vi "Boiler.vi"() -> ()   [LabVIEW 2020]
doc: "The VI \"Boiler\" is designed to simulate the operation of a boiler startup controller. This VI uses a state machine to control the states of its execution sequentially. Outside of the state machine are input variables that determine the maximum and minimum values required for events to take place as well the ability to name the event log file. Each state is indicated by the Boiler Status Indicators on the Front Panel and data collected from each state is written to the event log file. The states (with a short description of how to get to each state when applicable) are as follows and will repeat until the user presses STOP:\n\n1) Reset Controls and Indicators\n If state 10 has been executed: Wait 10s (or inputted value) for Shutdown and Purge to complete\n2) Start (Application Run)\n3) Reset Lockout\n \"Run Interlock\" ON and\n \"Boiler Reset\" ON\n4) Pre-Purge\n \"Start Sequence\" is ON\n5) Pre-Purge (continued)\n Wait 10 s (or inputted value) for Pre-Purge to complete\n6) Ignition (Ignite Pilot)\n \"Pilot\" is ON\n7) Prove the Pilot\n Flame Sensor Value (%) > 30 (or inputted minimum value)\n8) Start and Run\n Forced Draft Fan ON\n9) Start and run (continued)\n Fuel Valve Position > 10 (or inputted minimum value)\n10) Shutdown and Purge\n Run Interlock OFF or\n Forced Draft Fan OFF or\n Shutdown ON or\n Fuel Valve Position > 75 (or inputted maximum value) or\n Fuel Valve Position < 10 (or inputted minimum value)"
uses:
  Controls/Boiler Controls.ctl
  Controls/Boiler Simulation Controls.ctl
  Controls/Boiler Status Indicators.ctl
  Boiler States.ctl
panel:
  in  "stop":bool
  out "Boiler Status Indicators":T1 {"Time Count" format="%.2g"}
  in  "Boiler Simulation Controls":T2 {"Flame Sensor Value (%)" min=0.0 max=100.0 scale=0.0..100.0}
  in  "Boiler Controls":T3 {"Fuel Valve Position" min=0.0 max=100.0 scale=0.0..100.0 scale format="%.2f"}
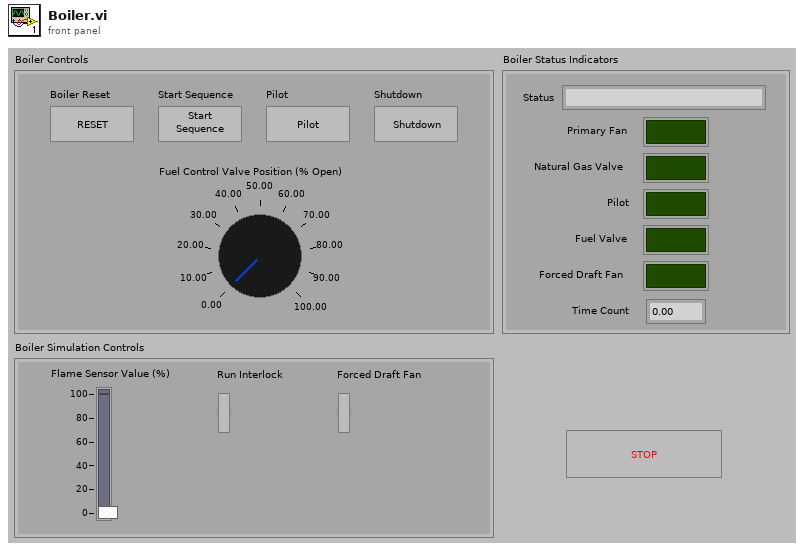
[diagram p1: front panel]
types:
  T1 = typedef "Boiler Status Indicators.ctl" = cluster{"Status":string, "Primary Fan":bool, "Natural Gas Valve":bool, "Pilot":bool, "Fuel Valve":bool, "Forced Draft Fan":bool, "Time Count":dbl}
  T2 = typedef "Boiler Simulation Controls.ctl" = cluster{"Flame Sensor Value (%)":dbl, "Run Interlock":bool, "Forced Draft Fan":bool}
  T3 = typedef "Boiler Controls.ctl" = cluster{"Boiler Reset":bool, "Start Sequence":bool, "Pilot":bool, "Shutdown":bool, "Fuel Valve Position":dbl}
  T4 = typedef "Boiler States.ctl" = enum16{"Reset Controls and Indicators", "Start (Application Run)", "Reset Lockout", "Pre-Purge", "Pre-Purge (continued)", "Ignition (Ignite Pilot)", "Prove the Pilot", "Start and Run", "Start and Run (continued)", "Shutdown and Purge"}
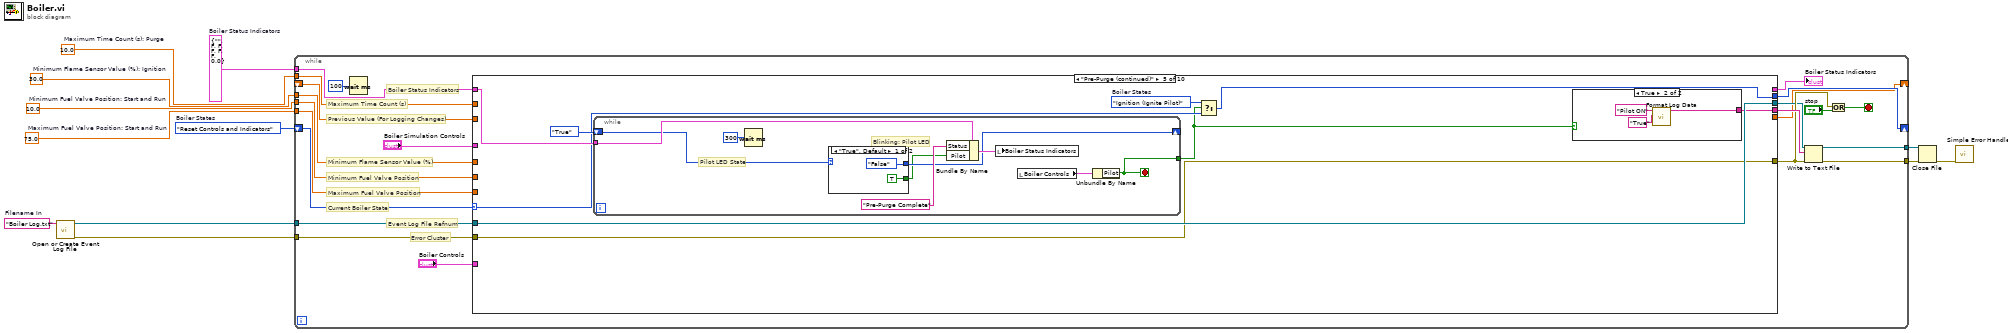
[diagram p0: block diagram]
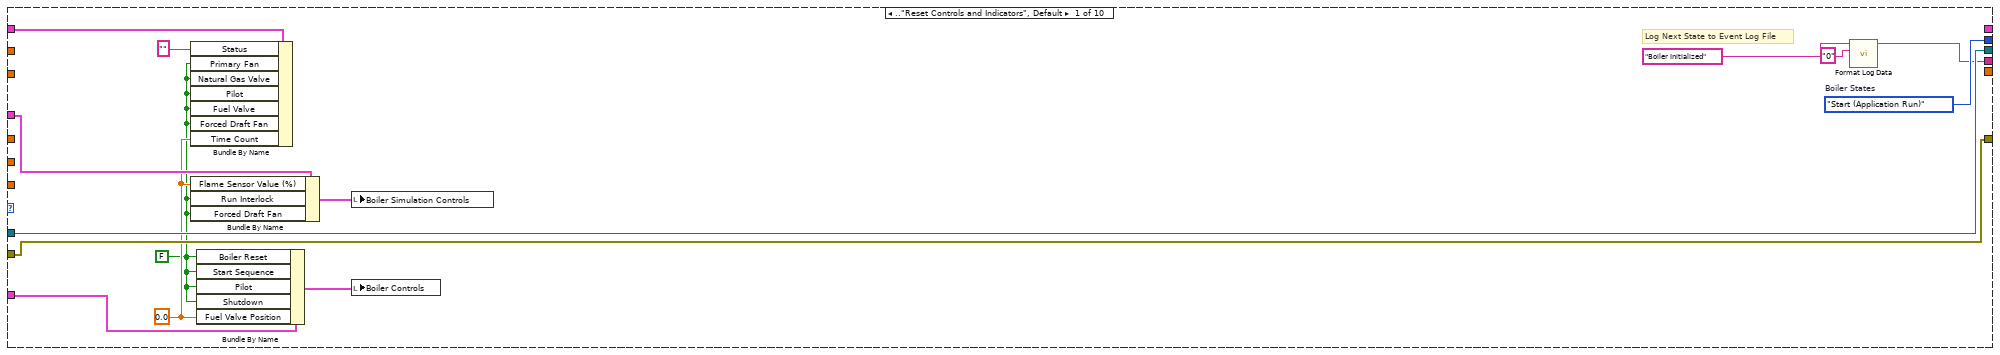
[diagram p2: hidden frame]
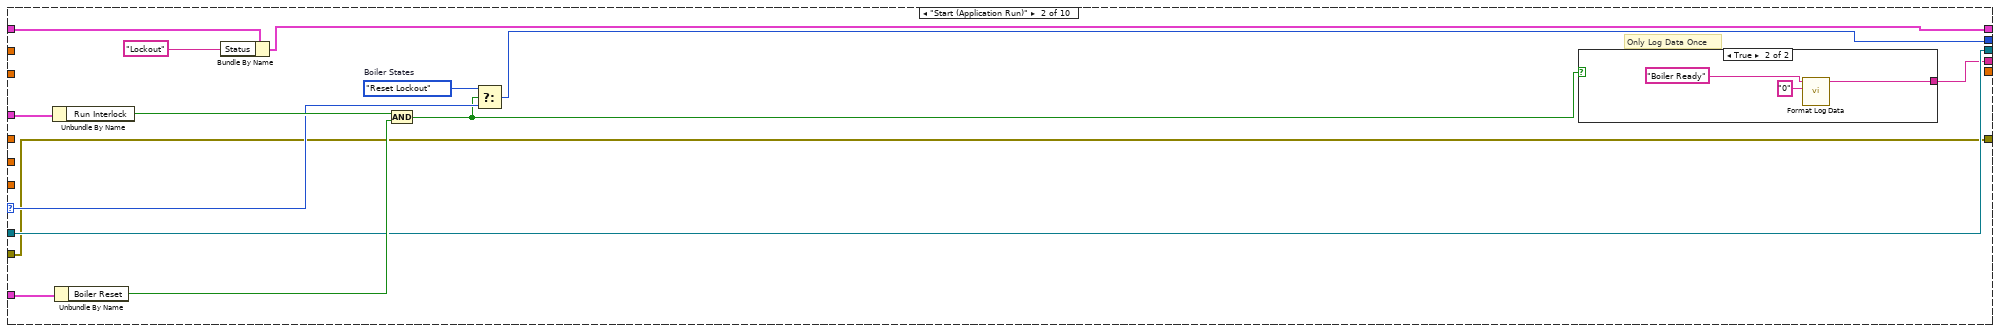
[diagram p3: hidden frame]
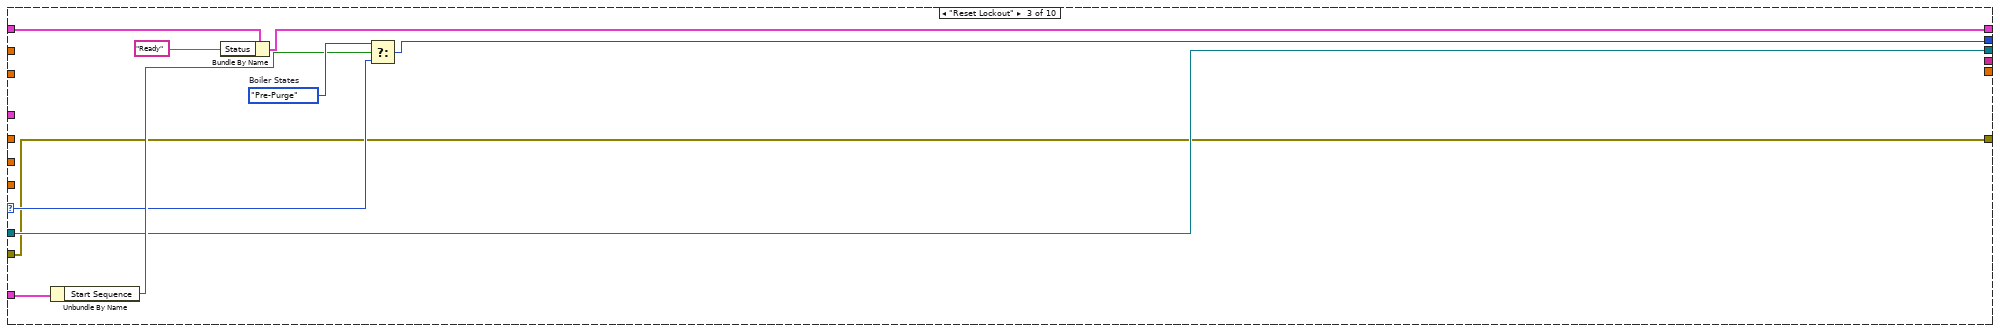
[diagram p5: hidden frame]
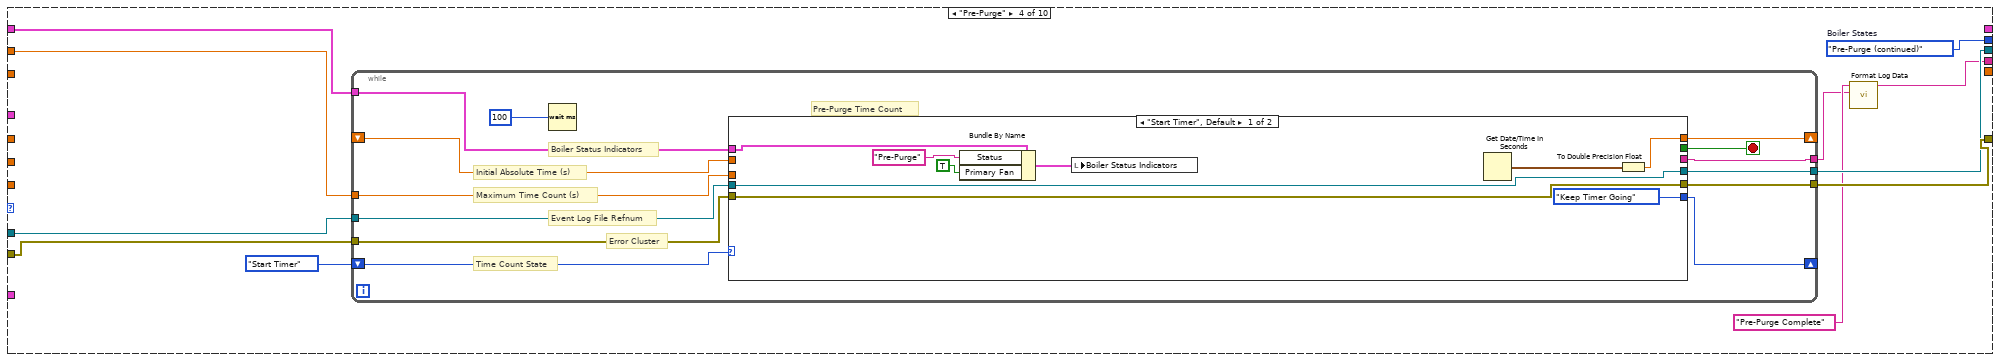
[diagram p6: hidden frame]
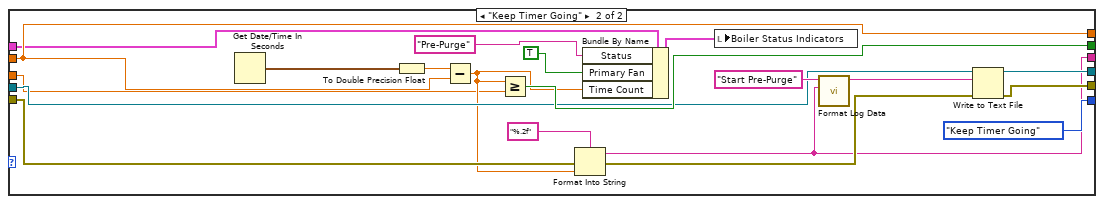
[diagram p7: hidden frame]
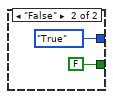
[diagram p9: hidden frame]
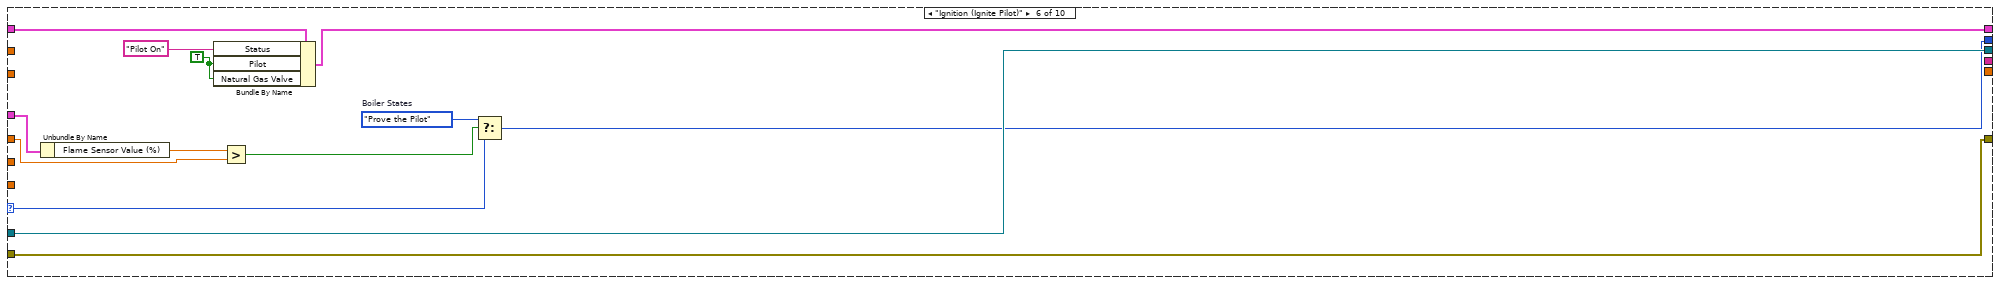
[diagram p10: hidden frame]
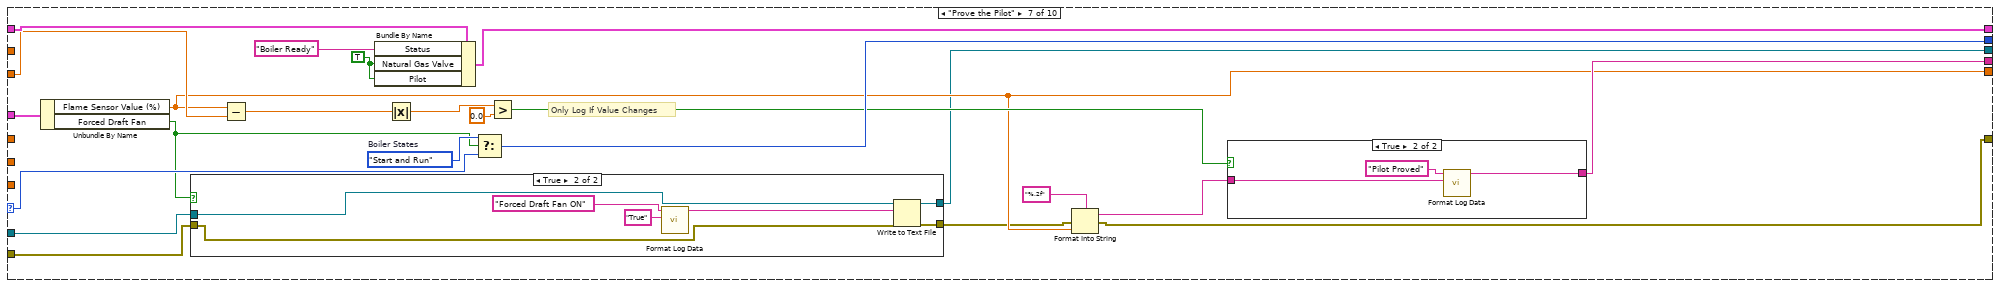
[diagram p11: hidden frame]
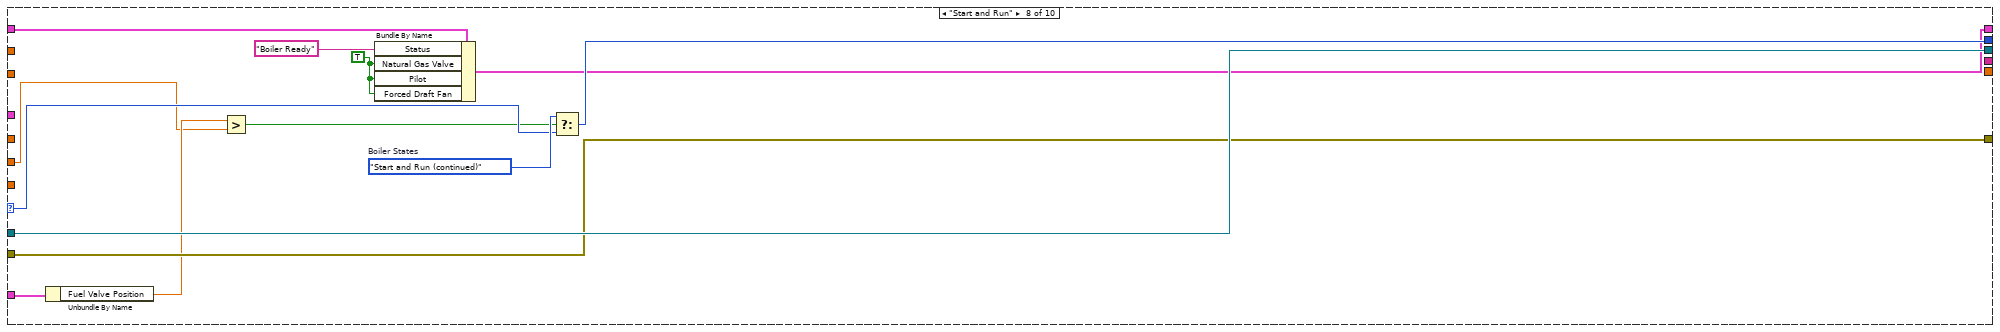
[diagram p14: hidden frame]
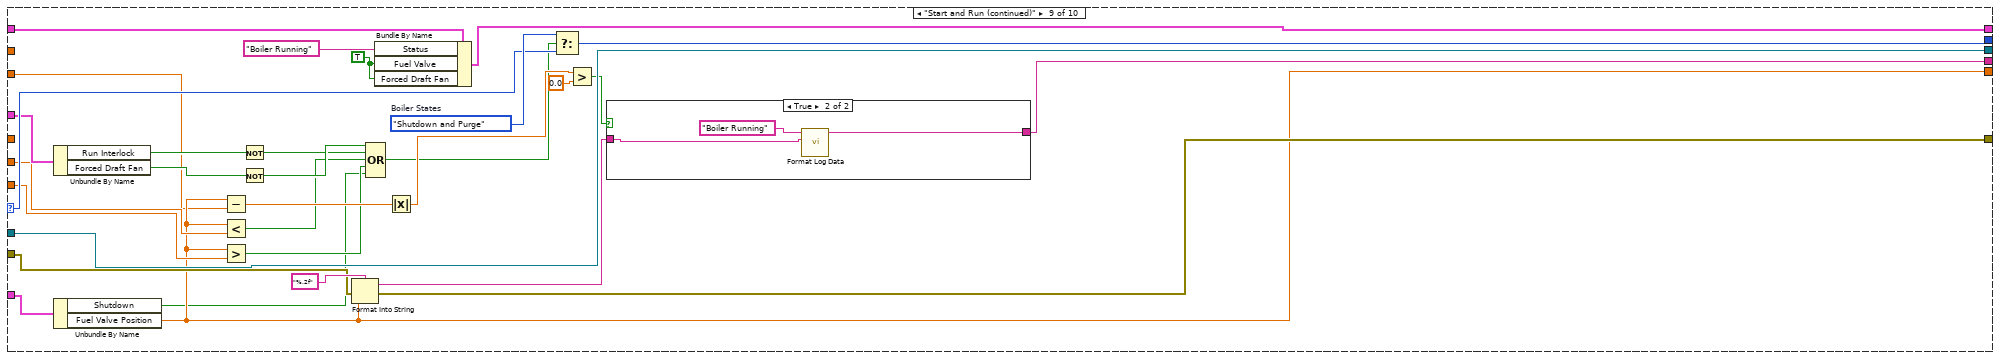
[diagram p15: hidden frame]
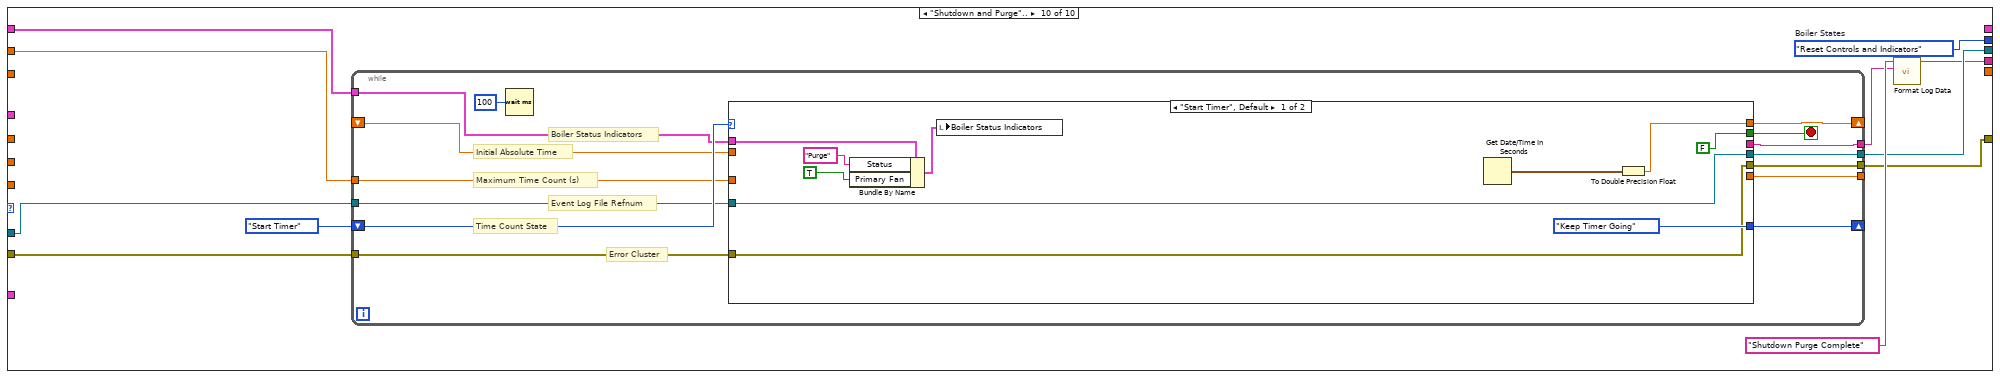
[diagram p17: hidden frame]
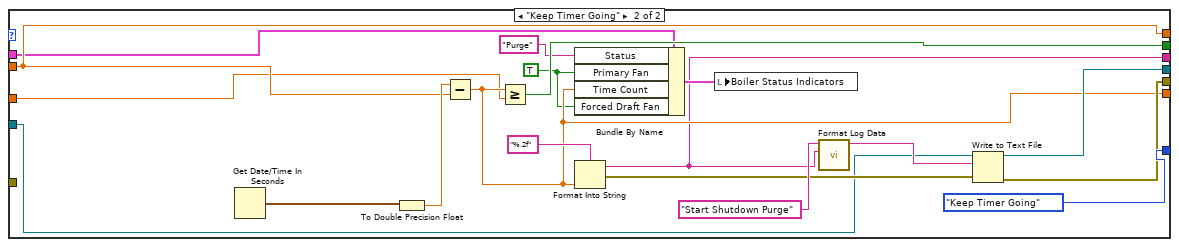
[diagram p18: hidden frame]
diagram:
  w1 = 75.0  # Maximum Fuel Valve Position: Start and Run
  w2 = 10.0  # Minimum Fuel Valve Position: Start and Run
  w3 = 30.0  # Minimum Flame Sensor Value (%): Ignition
  w4 = 10.0  # Maximum Time Count (s): Purge
  w5 = "Boiler Log.txt"  # Filename In
  w12 = T1 {"Status"="", "Primary Fan"=FALSE, "Natural Gas Valve"=FALSE, "Pilot"=FALSE, "Fuel Valve"=FALSE, "Forced Draft Fan"=FALSE, "Time Count"=0.0}  # Boiler Status Indicators
  w6 = Boiler_States."Reset Controls and Indicators"  # Boiler States
  n1 = call "Open or Create Event Log File.vi"("Filename In"=w5) -> ("error out"=w7:errorcluster, "refnum out"=w8:refnum<file>)  [unwired: 9 in]
  n2 = while {
    tunnel: w12 -> [w19]
    tunnel: [w29] -> w11
    tunnel: [w28] -> w10
    shift-right: [w27] -> _
    shift-left: w6 -> [w33]
    tunnel: w8 -> [w21]
    tunnel: w7 -> [w22]
    tunnel: w4 -> [w18]
    tunnel: w3 -> [w17]
    tunnel: w2 -> [w16]
    tunnel: w1 -> [w15]
    shift-right: [w14] -> _
    shift-left: _ -> [w13]
    stop <- w25 stop-if-true
    # "Previous Value (For Logging Changes)"
    # "Maximum Fuel Valve Position"
    # "Minimum Fuel Valve Position"
    # "Minimum Flame Sensor Value (%)"
    # "Maximum Time Count (s)"
    # "Boiler Status Indicators"
    # "Error Cluster"
    # "Event Log File Refnum"
    # "Current Boiler State"
    n3 = Wait (ms)(milliseconds to wait=u32 100) -> ()  [unwired: 1 out]
    n4 = case shown="\"Pre-Purge (continued)\"" w33 {
      selector: w33 -> [_ w53 w68 _ w135 w159 w180 w212 w234 _]
      tunnel: "Boiler Simulation Controls" -> [w45 w58 _ _ _ w157 w185 _ w233 _]
      tunnel: "Boiler Controls" -> [w43 w56 w70 _ _ _ _ w208 w232 _]
      tunnel: [_ w61 w74 _ _ w165 w189 w202 w244 _] -> w30
      tunnel: w19 -> [w41 w62 w75 w81 w137 w166 w188 w214 w245 w258]
      tunnel: [w48 w54 w71 w80 w133 w158 w179 w211 w235 w257] -> w27
      tunnel: [w35 w49 _ w77 w129 _ w186 _ w242 w251] -> w24
      tunnel: [w46 w51 w66 w85 w131 w162 w183 w209 w238 w253] -> w23
      tunnel: w22 -> [w46 w51 w66 w84 w131 w162 w170 w209 w239 w254]
      tunnel: w21 -> [w47 w52 w67 w83 w132 w161 w169 w210 w241 w255]
      tunnel: [w47 w52 w67 w82 w132 w161 w168 w210 w241 w252] -> w20
      tunnel: w18 -> [_ _ _ w76 _ _ _ _ _ w249]
      tunnel: w17 -> [_ _ _ _ _ w154 _ _ _ _]
      tunnel: w16 -> [_ _ _ _ _ _ _ w203 w228 _]
      tunnel: w15 -> [_ _ _ _ _ _ _ _ w227 _]
      tunnel: [_ _ _ _ _ _ w172 _ w226 _] -> w14
      tunnel: w13 -> [_ _ _ _ _ _ w173 _ w225 _]
      frame .."Reset Controls and Indicators", Default {
        w38 = FALSE ("Run Interlock")
        w39 = 0.0 ("Flame Sensor Value (%)")
        w48 = Boiler_States."Start (Application Run)"  # Boiler States
        # "Log Next State to Event Log File"
        n5 = Bundle By Name(cluster=w41, "Status"="", "Primary Fan"=w38, "Natural Gas Valve"=w38, "Pilot"=w38, "Fuel Valve"=w38, "Forced Draft Fan"=w38, "Time Count"=w39) -> ()  [unwired: 1 out]
        n6 = Bundle By Name(cluster=w45, "Flame Sensor Value (%)"=w39, "Run Interlock"=w38, "Forced Draft Fan"=w38) -> (w44:T2)
        n7 = Bundle By Name(cluster=w43, "Boiler Reset"=w38, "Start Sequence"=w38, "Pilot"=w38, "Shutdown"=w38, "Fuel Valve Position"=w39) -> (w42:T3)
        n8 = local write "Boiler Simulation Controls"(w44) -> ()
        n9 = local write "Boiler Controls"(w42) -> ()
        n10 = call "Format Log Data.vi"("Event Data String:"="0", "Event String:"="Boiler Initialized") -> ("Formatted Log Data"=w35:string)  [unwired: 9 in]
      }
      frame "Start (Application Run)" {
        w59 = Boiler_States."Reset Lockout"  # Boiler States
        # "Only Log Data Once"
        n11 = Unbundle By Name(w58) -> ("Run Interlock"=w57:bool)
        n12 = Unbundle By Name(w56) -> ("Boiler Reset"=w55:bool)
        n13 = Bundle By Name(cluster=w62, "Status"="Lockout") -> (w61:T1)
        n14 = And(x=w57, y=w55) -> (x .and. y?=w50:bool)
        n15 = Select(t=w59, s=w50, f=w53) -> (s? t:f=w54:T4)
        n16 = case shown="True" w50 {
          tunnel: [_ w63] -> w49
          frame False {
          }
          frame True {
            n17 = call "Format Log Data.vi"("Event Data String:"="0", "Event String:"="Boiler Ready") -> ("Formatted Log Data"=w63:string)  [unwired: 9 in]
          }
        }
      }
      frame "Reset Lockout" {
        w72 = Boiler_States."Pre-Purge"  # Boiler States
        n18 = Unbundle By Name(w70) -> ("Start Sequence"=w69:bool)
        n19 = Bundle By Name(cluster=w75, "Status"="Ready") -> (w74:T1)
        n20 = Select(t=w72, s=w69, f=w68) -> (s? t:f=w71:T4)
      }
      frame "Pre-Purge" {
        w80 = Boiler_States."Pre-Purge (continued)"  # Boiler States
        n21 = while {
          tunnel: w81 -> [w99]
          shift-right: [w96] -> _
          shift-left: enum16{"Start Timer", "Keep Timer Going"}."Start Timer" -> [w97]
          shift-right: [w95] -> _
          shift-left: _ -> [w94]
          tunnel: [w92] -> w85
          tunnel: w84 -> [w91]
          tunnel: w83 -> [w90]
          tunnel: [w89] -> w82
          tunnel: [w88] -> w78
          tunnel: w76 -> [w87]
          stop <- w93 stop-if-true
          # "Pre-Purge Time Count"
          # "Maximum Time Count (s)"
          # "Boiler Status Indicators"
          # "Initial Absolute Time (s)"
          # "Error Cluster"
          # "Time Count State"
          # "Event Log File Refnum"
          n22 = Wait (ms)(milliseconds to wait=u32 100) -> ()  [unwired: 1 out]
          n23 = case shown="\"Start Timer\", Default" w97 {
            tunnel: w99 -> [w101 w114]
            tunnel: [enum16{"Start Timer", "Keep Timer Going"}."Keep Timer Going" enum16{"Start Timer", "Keep Timer Going"}."Keep Timer Going"] -> w96
            tunnel: [w106 w124] -> w95
            tunnel: w94 -> [_ w124]
            tunnel: [_ w125] -> w93
            tunnel: [w104 w120] -> w92
            tunnel: w91 -> [w104 w117]
            tunnel: w90 -> [w105 w119]
            tunnel: [w105 w118] -> w89
            tunnel: [_ w110] -> w88
            tunnel: w87 -> [_ w109]
            frame "Start Timer", Default {
              n24 = Bundle By Name(cluster=w101, "Status"="Pre-Purge", "Primary Fan"=TRUE) -> (w100:T1)
              n25 = local write "Boiler Status Indicators"(w100) -> ()
              n26 = Get Date/Time In Seconds() -> (seconds since 1Jan1904=w107:timestamp)
              n27 = To Double Precision Float(number=w107) -> (double precision float=w106:dbl)
            }
            frame "Keep Timer Going" {
              n28 = Get Date/Time In Seconds() -> (seconds since 1Jan1904=w127:timestamp)
              n29 = To Double Precision Float(number=w127) -> (double precision float=w126:dbl)
              n30 = Subtract(x=w126, y=w124) -> (x-y=w111:dbl)
              n31 = Greater Or Equal?(x=w111, y=w109) -> (x >= y?=w125:bool)
              n32 = Format Into String "Format Into String"(format string="%.2f", error in=w117, w111) -> (resulting string=w110:string, error out=w116:errorcluster)  [unwired: 1 in]
              n33 = Bundle By Name(cluster=w114, "Status"="Pre-Purge", "Primary Fan"=TRUE, "Time Count"=w111) -> (w128:T1)
              n34 = local write "Boiler Status Indicators"(w128) -> ()
              n35 = call "Format Log Data.vi"("Event Data String:"=w110, "Event String:"="Start Pre-Purge") -> ("Formatted Log Data"=w121:string)  [unwired: 9 in]
              n36 = Write to Text File(file (use dialog)=w119, text=w121, error in=w116) -> (refnum out=w118:refnum<file>, error out=w120:errorcluster)  [unwired: 1 in, 1 out]
            }
          }
        }
        n37 = call "Format Log Data.vi"("Event Data String:"=w78, "Event String:"="Pre-Purge Complete") -> ("Formatted Log Data"=w77:string)  [unwired: 9 in]
      }
      frame "Pre-Purge (continued)" {
        w134 = Boiler_States."Ignition (Ignite Pilot)"  # Boiler States
        n38 = while {
          tunnel: w137 -> [w148]
          shift-right: [w144] -> _
          shift-left: enum16{"False", "True"}."True" -> [w145]
          tunnel: [w141] -> w130
          stop <- w141 stop-if-true
          # "Pilot LED State"
          # "Blinking: Pilot LED"
          n39 = Wait (ms)(milliseconds to wait=u32 300) -> ()  [unwired: 1 out]
          n40 = case shown="\"True\", Default" w145 {
            tunnel: [enum16{"False", "True"}."False" enum16{"False", "True"}."True"] -> w144
            tunnel: [TRUE FALSE] -> w143
            frame "True", Default {
            }
            frame "False" {
            }
          }
          n41 = Bundle By Name(cluster=w148, "Status"="Pre-Purge Complete", "Pilot"=w143) -> (w147:T1)
          n42 = local write "Boiler Status Indicators"(w147) -> ()
          n43 = local read "Boiler Controls"() -> (w142:T3)
          n44 = Unbundle By Name(w142) -> ("Pilot"=w141:bool)
        }
        n45 = Select(t=w134, s=w130, f=w135) -> (s? t:f=w133:T4)
        n46 = case shown="True" w130 {
          tunnel: [_ w138] -> w129
          frame False {
          }
          frame True {
            n47 = call "Format Log Data.vi"("Event Data String:"="True", "Event String:"="Pilot ON") -> ("Formatted Log Data"=w138:string)  [unwired: 9 in]
          }
        }
      }
      frame "Ignition (Ignite Pilot)" {
        w160 = Boiler_States."Prove the Pilot"  # Boiler States
        w163 = TRUE ("Natural Gas Valve")
        n48 = Unbundle By Name(w157) -> ("Flame Sensor Value (%)"=w156:dbl)
        n49 = Bundle By Name(cluster=w166, "Status"="Pilot On", "Pilot"=w163, "Natural Gas Valve"=w163) -> (w165:T1)
        n50 = Greater?(x=w156, y=w154) -> (0:w155:bool)
        n51 = Select(t=w160, s=w155, f=w159) -> (s? t:f=w158:T4)
      }
      frame "Prove the Pilot" {
        w178 = TRUE ("Natural Gas Valve")
        w181 = Boiler_States."Start and Run"  # Boiler States
        # "Only Log If Value Changes"
        n52 = Unbundle By Name(w185) -> ("Flame Sensor Value (%)"=w172:dbl, "Forced Draft Fan"=w171:bool)
        n53 = case shown="True" w171 {
          tunnel: w170 -> [w191 w196]
          tunnel: w169 -> [w190 w194]
          tunnel: [w190 w193] -> w168
          tunnel: [w191 w192] -> w167
          frame False {
          }
          frame True {
            n54 = call "Format Log Data.vi"("Event Data String:"="True", "Event String:"="Forced Draft Fan ON") -> ("Formatted Log Data"=w195:string)  [unwired: 9 in]
            n55 = Write to Text File(file (use dialog)=w194, text=w195, error in=w196) -> (refnum out=w193:refnum<file>, error out=w192:errorcluster)  [unwired: 1 in, 1 out]
          }
        }
        n56 = Subtract(x=w172, y=w173) -> (x-y=w177:dbl)
        n57 = Bundle By Name(cluster=w188, "Status"="Boiler Ready", "Natural Gas Valve"=w178, "Pilot"=w178) -> (w189:T1)
        n58 = Absolute Value(x=w177) -> (abs(x)=w176:dbl)
        n59 = Select(t=w181, s=w171, f=w180) -> (s? t:f=w179:T4)
        n60 = Greater?(x=w176, y=0.0) -> (0:w174:bool)
        n61 = Format Into String "Format Into String"(format string="%.2f", error in=w167, w172) -> (resulting string=w182:string, error out=w183:errorcluster)  [unwired: 1 in]
        n62 = case shown="True" w174 {
          tunnel: [_ w201] -> w186
          tunnel: w182 -> [_ w199]
          frame False {
          }
          frame True {
            n63 = call "Format Log Data.vi"("Event Data String:"=w199, "Event String:"="Pilot Proved") -> ("Formatted Log Data"=w201:string)  [unwired: 9 in]
          }
        }
      }
      frame "Start and Run" {
        w213 = Boiler_States."Start and Run (continued)"  # Boiler States
        w205 = TRUE ("Forced Draft Fan")
        n64 = Unbundle By Name(w208) -> ("Fuel Valve Position"=w207:dbl)
        n65 = Greater?(x=w207, y=w203) -> (0:w206:bool)
        n66 = Bundle By Name(cluster=w214, "Status"="Boiler Ready", "Natural Gas Valve"=w205, "Pilot"=w205, "Forced Draft Fan"=w205) -> (w202:T1)
        n67 = Select(t=w213, s=w206, f=w212) -> (s? t:f=w211:T4)
      }
      frame "Start and Run (continued)" {
        w236 = Boiler_States."Shutdown and Purge"  # Boiler States
        w230 = TRUE ("Fuel Valve")
        n68 = Unbundle By Name(w233) -> ("Run Interlock"=w229:bool, "Forced Draft Fan"=w231:bool)
        n69 = Unbundle By Name(w232) -> ("Shutdown"=w215:bool, "Fuel Valve Position"=w226:dbl)
        n70 = Subtract(x=w226, y=w225) -> (x-y=w224:dbl)
        n71 = Less?(x=w226, y=w228) -> (x < y?=w218:bool)
        n72 = Greater?(x=w226, y=w227) -> (0:w217:bool)
        n73 = Not(x=w229) -> (.not. x?=w219:bool)
        n74 = Not(x=w231) -> (.not. x?=w220:bool)
        n75 = Format Into String "Format Into String"(format string="%.2f", error in=w239, w226) -> (resulting string=w237:string, error out=w238:errorcluster)  [unwired: 1 in]
        n76 = Compound Arithmetic op=OR(w220, w219, w218, w217, w215) -> (w216:bool)
        n77 = Bundle By Name(cluster=w245, "Status"="Boiler Running", "Fuel Valve"=w230, "Forced Draft Fan"=w230) -> (w244:T1)
        n78 = Absolute Value(x=w224) -> (abs(x)=w223:dbl)
        n79 = Select(t=w236, s=w216, f=w234) -> (s? t:f=w235:T4)
        n80 = Greater?(x=w223, y=0.0) -> (0:w221:bool)
        n81 = case shown="True" w221 {
          tunnel: [_ w248] -> w242
          tunnel: w237 -> [_ w246]
          frame False {
          }
          frame True {
            n82 = call "Format Log Data.vi"("Event Data String:"=w246, "Event String:"="Boiler Running") -> ("Formatted Log Data"=w248:string)  [unwired: 9 in]
          }
        }
      }
      frame "Shutdown and Purge".. {
        w257 = Boiler_States."Reset Controls and Indicators"  # Boiler States
        n83 = while {
          shift-right: [w271] -> _
          shift-left: enum16{"Start Timer", "Keep Timer Going"}."Start Timer" -> [w272]
          shift-right: [w270] -> _
          shift-left: _ -> [w269]
          tunnel: [w267] -> w253
          tunnel: [w266] -> w252
          tunnel: [w265] -> _
          tunnel: w258 -> [w264]
          tunnel: w255 -> [w263]
          tunnel: w254 -> [w262]
          tunnel: [w261] -> w250
          tunnel: w249 -> [w260]
          stop <- w268 stop-if-true
          # "Initial Absolute Time"
          # "Maximum Time Count (s)"
          # "Event Log File Refnum"
          # "Time Count State"
          # "Error Cluster"
          # "Boiler Status Indicators"
          n84 = Wait (ms)(milliseconds to wait=u32 100) -> ()  [unwired: 1 out]
          n85 = case shown="\"Start Timer\", Default" w272 {
            tunnel: [enum16{"Start Timer", "Keep Timer Going"}."Keep Timer Going" enum16{"Start Timer", "Keep Timer Going"}."Keep Timer Going"] -> w271
            tunnel: [w281 w299] -> w270
            tunnel: w269 -> [_ w299]
            tunnel: [FALSE w300] -> w268
            tunnel: [w274 w296] -> w267
            tunnel: [w279 w295] -> w266
            tunnel: [_ w291] -> w265
            tunnel: w264 -> [w276 w289]
            tunnel: w263 -> [w279 w287]
            tunnel: w262 -> [w274 _]
            tunnel: [_ w286] -> w261
            tunnel: w260 -> [_ w284]
            frame "Start Timer", Default {
              n86 = Bundle By Name(cluster=w276, "Status"="Purge", "Primary Fan"=TRUE) -> (w275:T1)
              n87 = local write "Boiler Status Indicators"(w275) -> ()
              n88 = Get Date/Time In Seconds() -> (seconds since 1Jan1904=w282:timestamp)
              n89 = To Double Precision Float(number=w282) -> (double precision float=w281:dbl)
            }
            frame "Keep Timer Going" {
              w285 = TRUE ("Primary Fan")
              n90 = Get Date/Time In Seconds() -> (seconds since 1Jan1904=w302:timestamp)
              n91 = To Double Precision Float(number=w302) -> (double precision float=w301:dbl)
              n92 = Subtract(x=w301, y=w299) -> (x-y=w291:dbl)
              n93 = Greater Or Equal?(x=w291, y=w284) -> (x >= y?=w300:bool)
              n94 = Bundle By Name(cluster=w289, "Status"="Purge", "Primary Fan"=w285, "Time Count"=w291, "Forced Draft Fan"=w285) -> (w290:T1)
              n95 = Format Into String "Format Into String"(format string="%.2f", w291) -> (resulting string=w286:string, error out=w294:errorcluster)  [unwired: 2 in]
              n96 = local write "Boiler Status Indicators"(w290) -> ()
              n97 = call "Format Log Data.vi"("Event Data String:"=w286, "Event String:"="Start Shutdown Purge") -> ("Formatted Log Data"=w288:string)  [unwired: 9 in]
              n98 = Write to Text File(file (use dialog)=w287, text=w288, error in=w294) -> (refnum out=w295:refnum<file>, error out=w296:errorcluster)  [unwired: 1 in, 1 out]
            }
          }
        }
        n99 = call "Format Log Data.vi"("Event Data String:"=w250, "Event String:"="Shutdown Purge Complete") -> ("Formatted Log Data"=w251:string)  [unwired: 9 in]
      }
    }
    "Boiler Status Indicators" <- w30
    n100 = Write to Text File(file (use dialog)=w20, text=w24, error in=w23) -> (refnum out=w28:refnum<file>, error out=w29:errorcluster)  [unwired: 1 in, 1 out]
    n101 = Or(x=w23, y="stop") -> (x .or. y?=w25:bool)
  }
  n102 = Close File(refnum=w10, error in=w11) -> (error out=w9:errorcluster)  [unwired: 1 out]
  n103 = call <vilib>:"Simple Error Handler.vi"("error in (no error)"=w9) -> ()  [unwired: 4 in, 5 out]
